vi "UIRef.vi"(8 "error in":errorcluster, 11 "node in":refnum<class "TBM Configuration Node.lvclass">) -> (0 "error out":errorcluster, 2 "VI refnum":refnum<vi>, 3 "node out":refnum<class "TBM Configuration Node.lvclass">)   [LabVIEW 2013, in "PL Framework Configuration Tool.lvlib" / "TBM Configuration Node.lvclass"]
doc: "Stores the static reference to the UI of the node."
uses:
  TBM Configuration Node.lvclass
  <vilib>/NI/Configuration Framework/serializable node/NISE_CEF_serializable node.lvclass
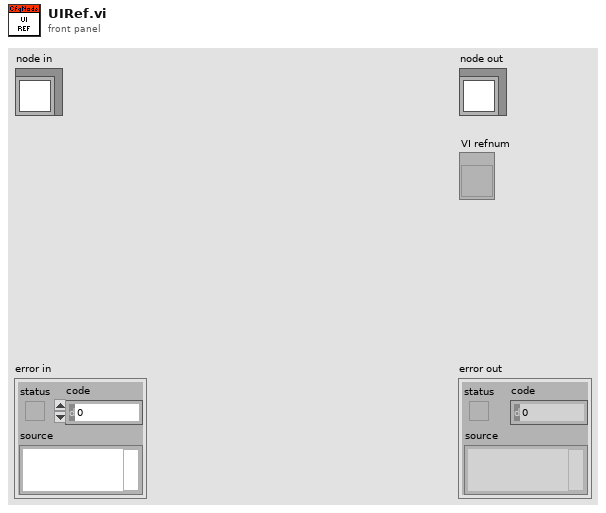
[diagram p1: front panel]
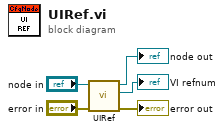
[diagram p0: block diagram]
diagram:
  n1 = call-parent "UIRef.vi"("error in"="error in", "node in"="node in") -> ("error out"=→"error out":errorcluster, "VI refnum"=→"VI refnum":refnum<vi>, "node out"=→"node out":refnum<class "TBM Configuration Node.lvclass">)  [unwired: 7 in]
